vi "Calibration Code for Sonar.vi"() -> ()   [LabVIEW 2014]
uses:
  <vilib>/Instr/_visa.llb/VISA Flush IO Buffer Mask.ctl
  <vilib>/Instr/_visa.llb/VISA Configure Serial Port (Instr).vi
  <vilib>/Utility/file.llb/Read From Spreadsheet File (DBL).vi
panel:
  out "Final Decision Array":dbl[](graph)
  in  "Avg":path
  in  "Min":path
  out "SubFinal Decision Array":dbl[](graph)
  out "Normalized Scan 1":dbl[](graph)
  out "Normalized Scan 2":dbl[](graph)
  out "error out":errorcluster
  out "Done":bool
  out "Position Out":i32
  out "Loop Number":i32
  out "Gauge":i32(knob)
  in  "stop 2":bool
  out "Sensor Head Position 2":i32
  out "THE WHALE IS AT:":i32
  out "Waveform Graph 2":dbl[](graph)
  in  "?":bool
  out "Stop Engaged 2":bool
  out "Blinky Light 2":bool
  out "read buffer 3":string
  out "return count 3":u32
  out "Distance, in 3":dbl
  out "Waveform Chart 4":dbl(graph)
  in  "Max":path
  out "Waveform Graph":dbl[](graph)
  out "error out 2":errorcluster
  in  "Motor Direction":bool
  in  "?":bool
  out "Stop Engaged":bool
  out "Blinky Light":bool
  out "Sensor Head Position":dbl
  out "Sensor Head Dial":dbl(knob) scale=-800.0..800.0
  out "read buffer 2":string
  out "return count 2":u32
  out "Distance, in 2":dbl
  out "Waveform Chart 3":dbl(graph)
  in  "stop":bool
  out "IR Distance Reading":dbl
  out "Find starting position?":bool
  in  "VISA resource name 2":refnum<visa-resource-name>="COM3"
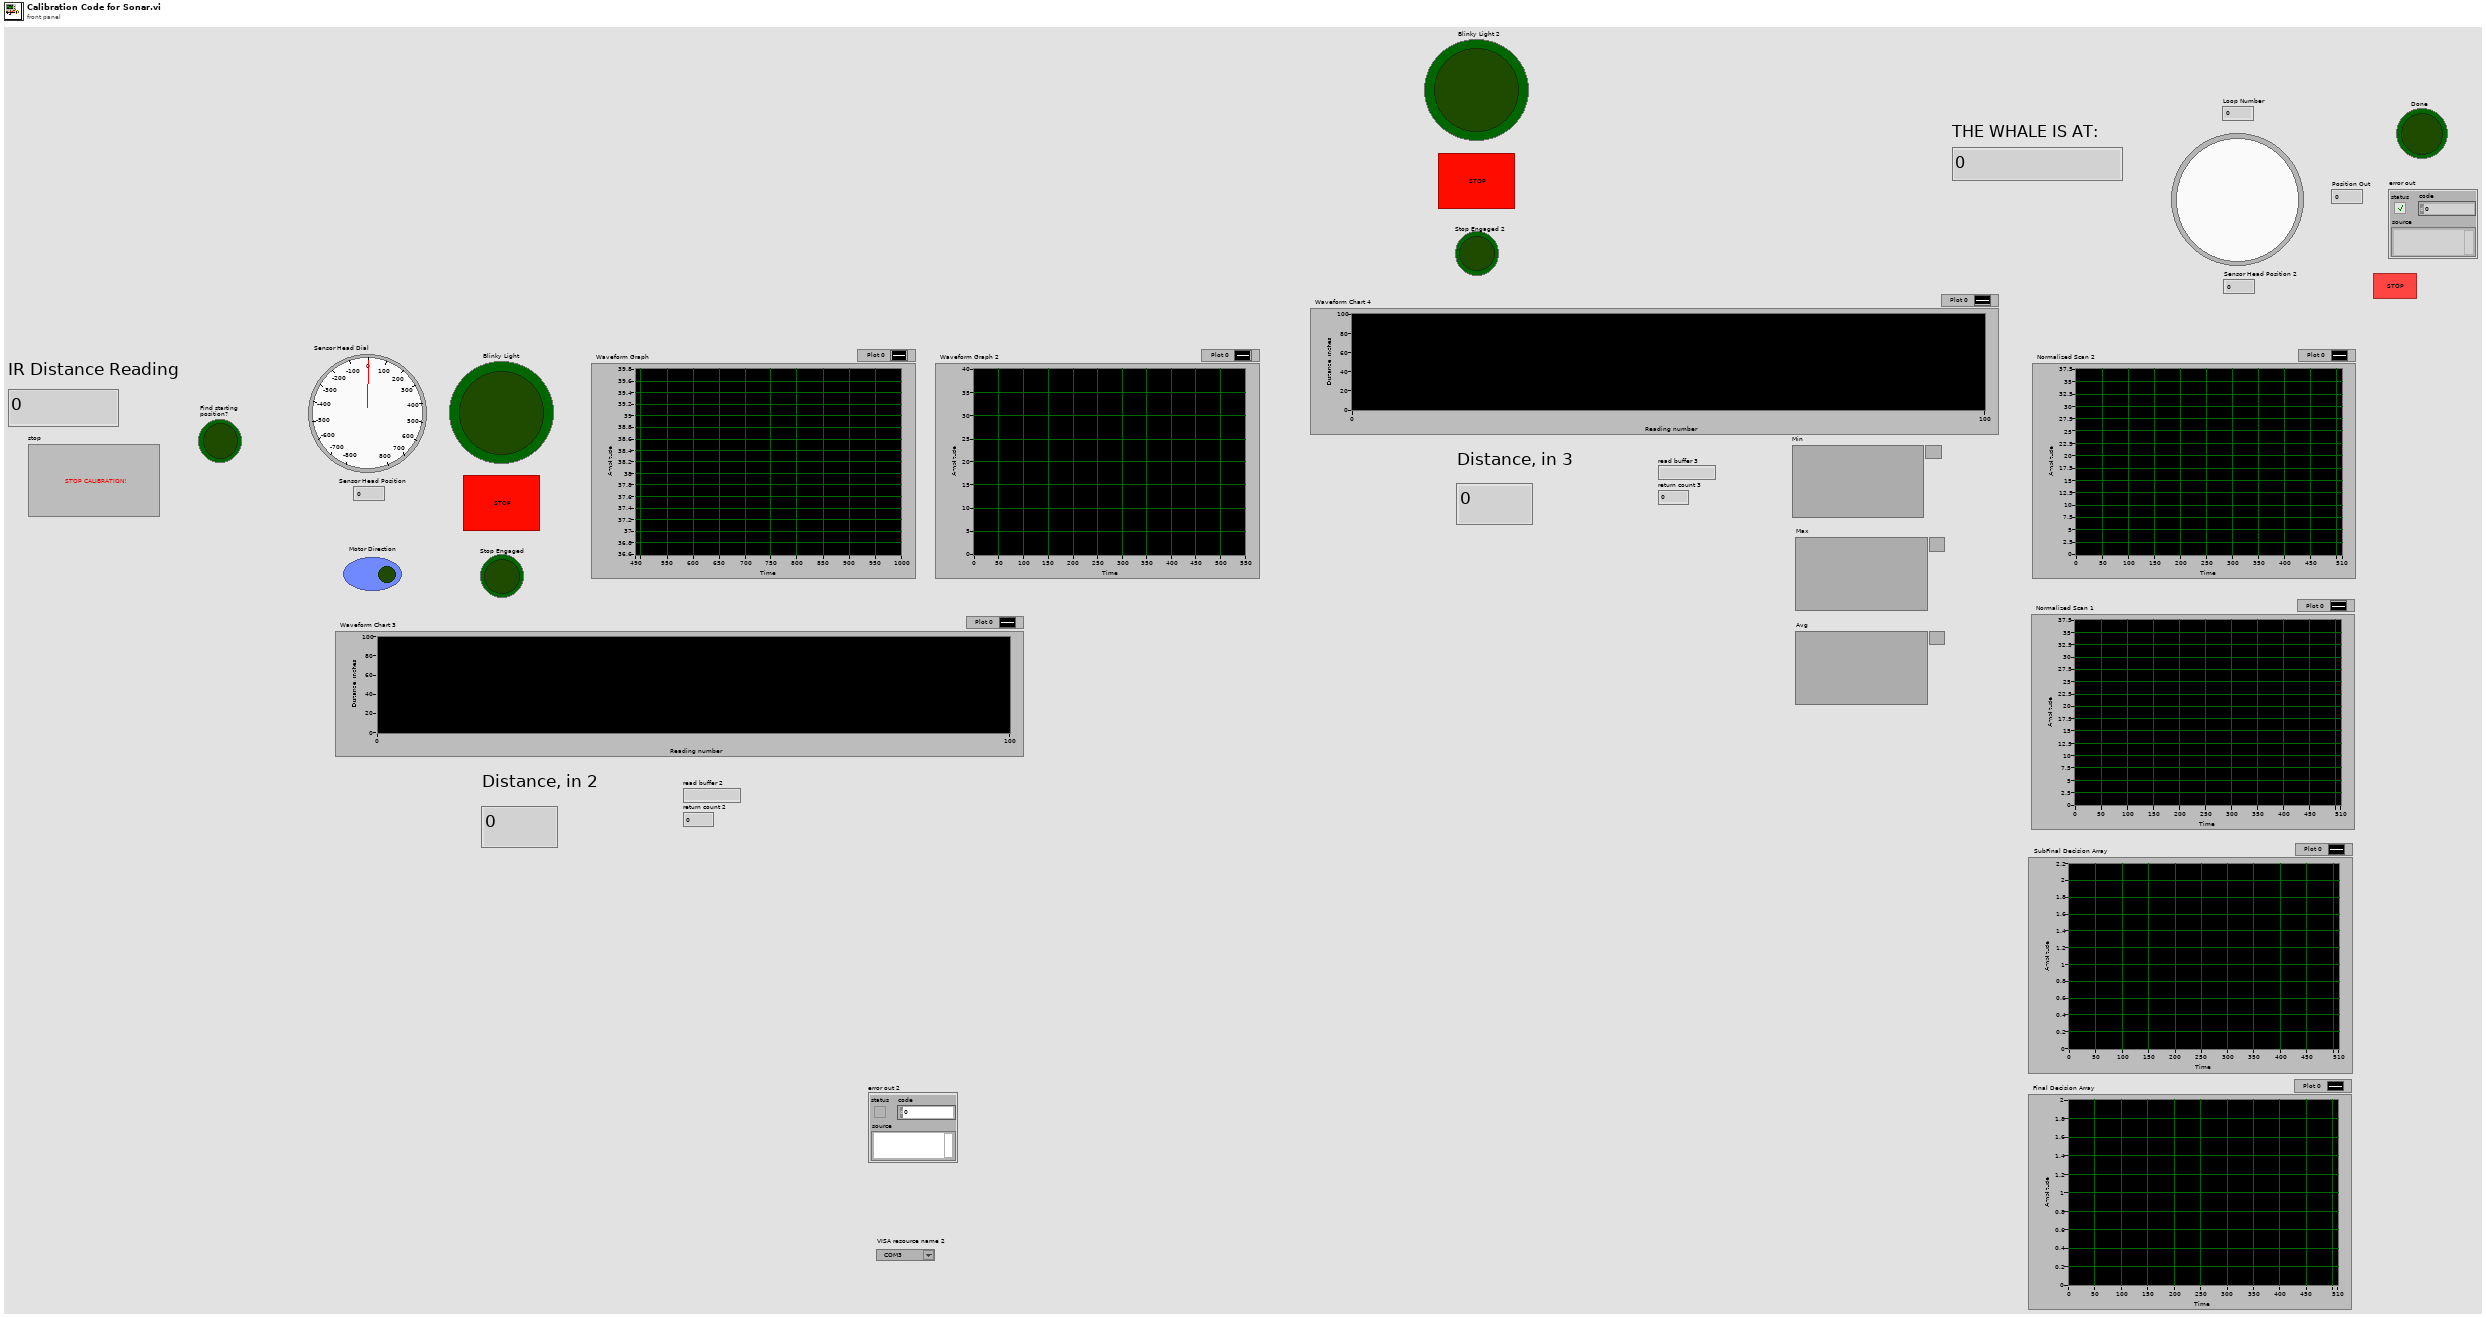
[diagram p1: front panel]
types:
  T1 = typedef "VISA Flush IO Buffer Mask.ctl" = u16
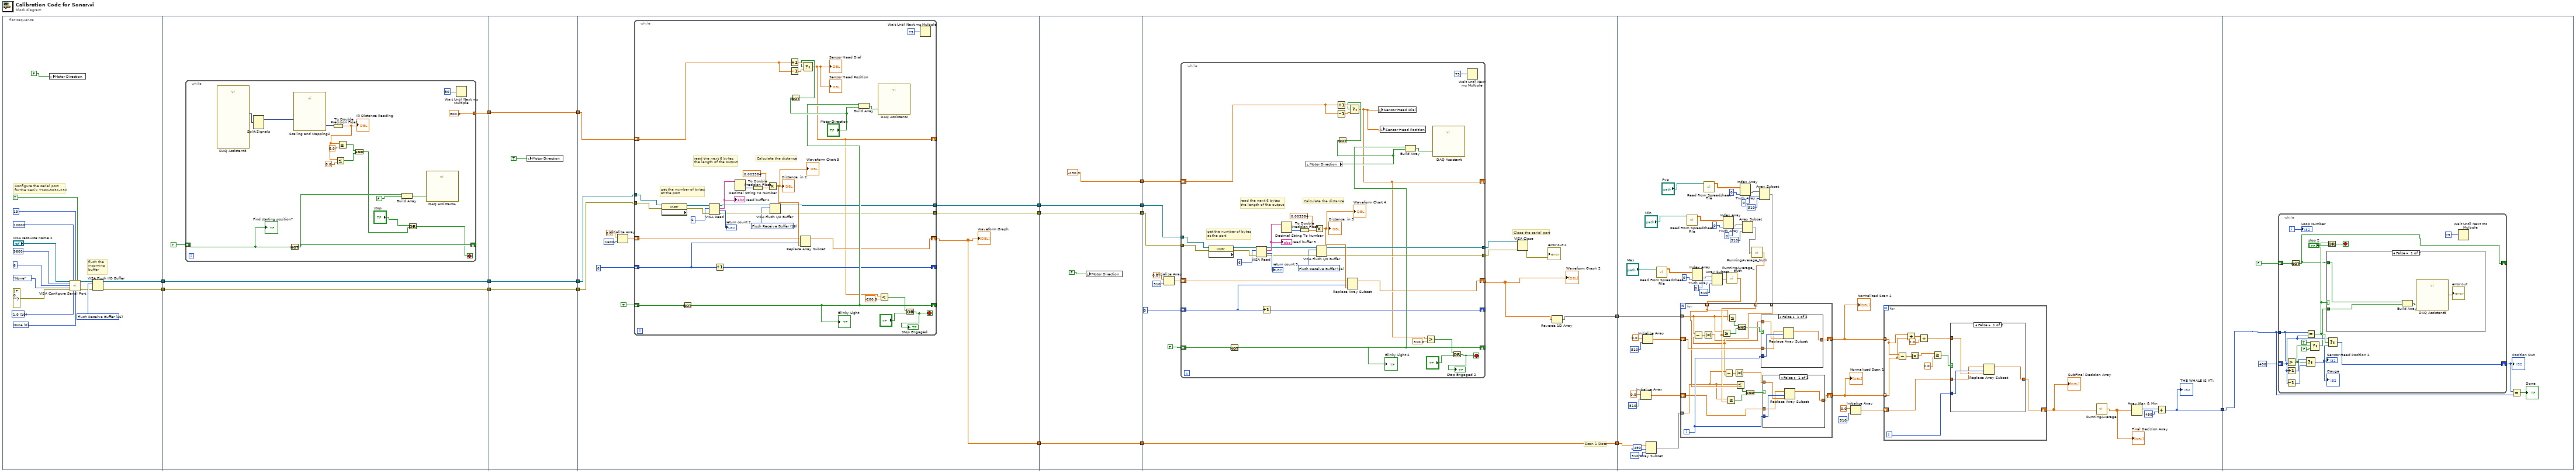
[diagram p0: block diagram]
diagram:
  n1 = flat-sequence {
    tunnel: [w21] -> w18
    tunnel: [w20] -> w17
    tunnel: w18 -> [w38]
    tunnel: w17 -> [w37]
    tunnel: [w35] -> w16
    tunnel: [w38] -> w15
    tunnel: [w37] -> w14
    tunnel: w16 -> [w59]
    tunnel: w15 -> [w58]
    tunnel: w14 -> [w57]
    tunnel: [w59] -> w13
    tunnel: [w58] -> w12
    tunnel: [w57] -> w11
    tunnel: w13 -> [w68]
    tunnel: w12 -> [w67]
    tunnel: w11 -> [w66]
    tunnel: [w62] -> w10
    tunnel: [w61] -> w8
    tunnel: [w60] -> w5
    tunnel: w10 -> [w109]
    tunnel: [w109] -> w9
    tunnel: w8 -> [w108]
    tunnel: [w108] -> w7
    tunnel: [-250.0] -> w6
    tunnel: w5 -> [w105]
    tunnel: [w105] -> w4
    tunnel: w9 -> [w117]
    tunnel: w7 -> [w116]
    tunnel: w6 -> [w115]
    tunnel: w4 -> [w114]
    tunnel: [w114] -> w3
    tunnel: [w110] -> w2
    tunnel: w3 -> [w201]
    tunnel: w2 -> [w199]
    tunnel: [w200] -> w1
    tunnel: w1 -> [w253]
    frame #0 {
      w24 = T1 16 items=["Flush Receive Buffer"=16, "Write Transmit Buffer to Device"=32, "Flush Receive Buffer (No I/O)"=64, "Flush Transmit Buffer"=128] ("Mask")
      w28 = u16 0 items=["None", "XON/XOFF", "RTS/CTS", "XON/XOFF & RTS/CTS", "DTR/DSR", "XON/XOFF & DTR/DSR"] ("flow control (0:none)")
      w30 = u16 10 items=["1.0"=10, "1.5"=15, "2.0"=20] ("stop bits (10: 1 bit)")
      # "flush the \nincoming \nbuffer"
      # "Configure the serial port\nfor the Senix TSPC-3031-232"
      n2 = local write "Motor Direction"(FALSE) -> ()
      n3 = call-poly "VISA Configure Serial Port"("VISA resource name"="VISA resource name 2", "timeout (10sec)"=u32 10000, "termination char\n(0xA = '\\n' = LF)"=u8 13 ("termination char\n(0xA = '\\n' = LF)"), "Enable Termination\nChar (T)"=TRUE ("Enable Termination\nChar (T)"), "baud rate (9600)"=u32 9600, "data bits (8)"=u16 8, "parity (0:none)"=enum16{"None", "Odd", "Even", "Mark", "Space"}."None", "error in (no error)"=errorcluster {"status"=FALSE, "code"=0, "source"=""}, "stop bits (10: 1 bit)"=w30, "flow control (0:none)"=w28) -> ("VISA resource name out"=w23:refnum<visa-resource-name>, "error out"=w22:errorcluster)  [unwired: 4 in]
      n4 = VISA Flush I/O Buffer(VISA resource name=w23, mask (16)=w24, error in (no error)=w22) -> (VISA resource name out=w21:refnum<visa-resource-name>, error out=w20:errorcluster)
    }
    frame #1 {
      n5 = while {
        tunnel: [800.0] -> w35
        shift-right: [w54] -> _
        shift-left: TRUE -> [w52]
        stop <- w41 stop-if-true
        n6 = call "DAQ Assistant3"() -> ("data"=w50:dynamicdata)  [unwired: 16 in, 3 out]
        n7 = Split Signals "Split Signals"(w50) -> (w51:dynamicdata)  [unwired: 5 in, 4 out]
        n8 = Not(x=w52) -> (.not. x?=w54:bool)
        n9 = call "Scaling and Mapping2"("Signals"=w51) -> ("Scaled Signals"=w45:dynamicdata)  [unwired: 9 in, 1 out]
        n10 = To Double Precision Float(number=w45) -> (double precision float=w44:dbl)
        "IR Distance Reading" <- w44
        n11 = Less Or Equal?(x=w44, y=8.0) -> (x <= y?=w46:bool)
        n12 = Greater Or Equal?(x=w44, y=6.0) -> (x >= y?=w47:bool)
        n13 = And(x=w47, y=w46) -> (x .and. y?=w42:bool)
        n14 = Build Array(w54, FALSE) -> (w55:bool[])
        n15 = Or(x="stop", y=w42) -> (x .or. y?=w41:bool)
        n16 = call "DAQ Assistant4"("data"=w55) -> ()  [unwired: 17 in, 2 out]
        n17 = Wait Until Next ms Multiple(millisecond multiple=50) -> ()  [unwired: 1 out]
        "Find starting position?" <- w52
      }
    }
    frame #2 {
      n18 = local write "Motor Direction"(TRUE) -> ()
    }
    frame #3 {
      n19 = Initialize Array(0.0 ("element"), 1600 ("dimension size")) -> (w69:dbl[])
      n20 = while {
        shift-right: [w71] -> _
        shift-left: w68 -> [w101]
        shift-right: [w82] -> _
        shift-left: TRUE -> [w96]
        tunnel: w67 -> [w81]
        tunnel: w66 -> [w80]
        shift-right: [w77] -> w60
        shift-left: w69 -> [w79]
        shift-right: [w76] -> _
        shift-left: 0 ("dimension size") -> [w78]
        tunnel: [w75] -> w61
        tunnel: [w74] -> w62
        stop <- w95 stop-if-true
        w85 = T1 16 items=["Flush Receive Buffer"=16, "Write Transmit Buffer to Device"=32, "Flush Receive Buffer (No I/O)"=64, "Flush Transmit Buffer"=128] ("Mask")
        # "Calculate the distance"
        # "read the next 6 bytes\nthe length of the output"
        # "get the number of bytes\nat the port"
        n21 = property class="Instr" props=["Serial Settings:Number of Bytes at Serial Port"](reference=w81, error in=w80) -> (reference out=w94:refnum<visa-resource-name>, error out=w93:errorcluster)  [unwired: 1 out]
        n22 = Not(x=w96) -> (.not. x?=w82:bool)
        "Blinky Light" <- w82
        n23 = VISA Read(VISA resource name=w94, byte count=u32 6, error in (no error)=w93) -> (VISA resource name out=w87:refnum<visa-resource-name>, read buffer=w91:string, return count=→"return count 2":u32, error out=w86:errorcluster)
        "read buffer 2" <- w91
        n24 = Increment(x=w78) -> (x+1=w76:i32)
        n25 = Decimal String To Number(string=w91) -> (number=w90:i32)  [unwired: 2 in, 1 out]
        n26 = To Double Precision Float(number=w90) -> (double precision float=w89:dbl)
        n27 = Multiply(x=0.003384, y=w89) -> (x*y=w83:dbl)
        "Distance, in 2" <- w83
        "Waveform Chart 3" <- w83
        n28 = VISA Flush I/O Buffer(VISA resource name=w87, mask (16)=w85, error in (no error)=w86) -> (VISA resource name out=w75:refnum<visa-resource-name>, error out=w74:errorcluster)
        n29 = Increment(x=w101) -> (x+1=w103:dbl)
        n30 = Decrement(x=w101) -> (x-1=w102:dbl)
        n31 = Not(x="Motor Direction") -> (.not. x?=w99:bool)
        n32 = Replace Array Subset(array=w79, new element=w83, index=w78) -> (w77:dbl[])
        n33 = Select(t=w103, s=w99, f=w102) -> (s? t:f=w71:dbl)
        "Sensor Head Position" <- w71
        "Sensor Head Dial" <- w71
        n34 = Build Array(w82, "Motor Direction") -> (w97:bool[])
        n35 = call "DAQ Assistant2"("data"=w97) -> ()  [unwired: 17 in, 2 out]
        n36 = Less?(x=w71, y=-200.0) -> (x < y?=w73:bool)
        n37 = Or(x=w73, y="?") -> (x .or. y?=w95:bool)
        "Stop Engaged" <- w95
        n38 = Wait Until Next ms Multiple(millisecond multiple=75) -> ()  [unwired: 1 out]
      }
      "Waveform Graph" <- w60
    }
    frame #4 {
      n39 = local write "Motor Direction"(FALSE) -> ()
    }
    frame #5 {
      # "Scan 1 Data"
      # "Close the serial port"
      n40 = Initialize Array(0.0 ("element"), 510 ("dimension size")) -> (w121:dbl[])
      n41 = while {
        shift-right: [w124] -> _
        shift-left: w115 -> [w154]
        shift-right: [w136] -> _
        shift-left: TRUE -> [w150]
        tunnel: w116 -> [w135]
        tunnel: w117 -> [w134]
        shift-right: [w131] -> w111
        shift-left: w121 -> [w133]
        shift-right: [w130] -> _
        shift-left: 0 ("dimension size") -> [w132]
        tunnel: [w129] -> w113
        tunnel: [w128] -> w112
        stop <- w149 stop-if-true
        w139 = T1 16 items=["Flush Receive Buffer"=16, "Write Transmit Buffer to Device"=32, "Flush Receive Buffer (No I/O)"=64, "Flush Transmit Buffer"=128] ("Mask")
        # "Calculate the distance"
        # "read the next 6 bytes\nthe length of the output"
        # "get the number of bytes\nat the port"
        n42 = property class="Instr" props=["Serial Settings:Number of Bytes at Serial Port"](reference=w135, error in=w134) -> (reference out=w148:refnum<visa-resource-name>, error out=w147:errorcluster)  [unwired: 1 out]
        n43 = Not(x=w150) -> (.not. x?=w136:bool)
        "Blinky Light 2" <- w136
        n44 = VISA Read(VISA resource name=w148, byte count=u32 6, error in (no error)=w147) -> (VISA resource name out=w141:refnum<visa-resource-name>, read buffer=w145:string, return count=→"return count 3":u32, error out=w140:errorcluster)
        "read buffer 3" <- w145
        n45 = Increment(x=w132) -> (x+1=w130:i32)
        n46 = Decimal String To Number(string=w145) -> (number=w144:i32)  [unwired: 2 in, 1 out]
        n47 = To Double Precision Float(number=w144) -> (double precision float=w143:dbl)
        n48 = local read "Motor Direction"() -> (w125:bool)
        n49 = Multiply(x=0.003384, y=w143) -> (x*y=w137:dbl)
        "Distance, in 3" <- w137
        "Waveform Chart 4" <- w137
        n50 = VISA Flush I/O Buffer(VISA resource name=w141, mask (16)=w139, error in (no error)=w140) -> (VISA resource name out=w129:refnum<visa-resource-name>, error out=w128:errorcluster)
        n51 = Increment(x=w154) -> (x+1=w156:dbl)
        n52 = Decrement(x=w154) -> (x-1=w155:dbl)
        n53 = Not(x=w125) -> (.not. x?=w152:bool)
        n54 = Replace Array Subset(array=w133, new element=w137, index=w132) -> (w131:dbl[])
        n55 = Select(t=w156, s=w152, f=w155) -> (s? t:f=w124:dbl)
        n56 = local write "Sensor Head Dial"(w124) -> ()
        n57 = local write "Sensor Head Position"(w124) -> ()
        n58 = Build Array(w136, w125) -> (w151:bool[])
        n59 = Greater?(x=w124, y=310.0) -> (0:w127:bool)
        n60 = call "DAQ Assistant"("data"=w151) -> ()  [unwired: 17 in, 2 out]
        n61 = Or(x=w127, y="?") -> (x .or. y?=w149:bool)
        "Stop Engaged 2" <- w149
        n62 = Wait Until Next ms Multiple(millisecond multiple=75) -> ()  [unwired: 1 out]
      }
      "Waveform Graph 2" <- w111
      n63 = VISA Close(VISA resource name=w113, error in (no error)=w112) -> (error out=→"error out 2":errorcluster)
      n64 = Reverse 1D Array(array=w111) -> (reversed array=w110:dbl[])
    }
    frame #6 {
      n65 = Initialize Array "Initialize Array"(0.0 ("element"), 510 ("dimension size")) -> (w187:dbl[])
      n66 = Initialize Array "Initialize Array"(0.0 ("element"), 510 ("dimension size")) -> (w190:dbl[])
      n67 = Array Subset(array=w201, index=490, length=510) -> (w196:dbl[])
      n68 = call-poly <vilib>:"Read From Spreadsheet File.vi"("file path (dialog if empty)"="Max") -> ("all rows"=w194:dbl[][])  [unwired: 6 in, 4 out]
      n69 = call-poly <vilib>:"Read From Spreadsheet File.vi"("file path (dialog if empty)"="Min") -> ("all rows"=w176:dbl[][])  [unwired: 6 in, 4 out]
      n70 = Index Array "Truth Array"(array=w194, index (col)=0 ("index")) -> (element=w181:dbl[])  [unwired: 1 in]
      n71 = call-poly <vilib>:"Read From Spreadsheet File.vi"("file path (dialog if empty)"="Avg") -> ("all rows"=w170:dbl[][])  [unwired: 6 in, 4 out]
      n72 = Array Subset(array=w181, index=0, length=510) -> (w161:dbl[])
      n73 = Index Array "Truth Array"(array=w176, index (col)=0 ("index")) -> (element=w174:dbl[])  [unwired: 1 in]
      n74 = call "RunningAverage_truth.vi"("Input Decision Array"=w161) -> ("Output Decision Array"=w160:dbl[])
      n75 = Index Array "Truth Array"(array=w170, index (col)=0 ("index")) -> (element=w168:dbl[])  [unwired: 1 in]
      n76 = Array Subset(array=w174, index=0, length=510) -> (w159:dbl[])
      n77 = call "RunningAverage_truth.vi"("Input Decision Array"=w159) -> ("Output Decision Array"=w158:dbl[])
      n78 = Array Subset(array=w168, index=0, length=510) -> (w164:dbl[])
      n79 = for {
        tunnel: w199 -> [w221] mode=indexing
        tunnel: w160 -> [w233] mode=indexing
        shift-right: [w237] -> w178
        shift-left: w190 -> [w238]
        tunnel: w196 -> [w223] mode=indexing
        shift-right: [w234] -> w177
        shift-left: w187 -> [w235]
        tunnel: w158 -> [w232] mode=indexing
        tunnel: w164 -> [w220] mode=indexing
        i -> [w236]
        n80 = Subtract(x=w221, y=w220) -> (x-y=w225:dbl)
        n81 = Absolute Value(x=w225) -> (abs(x)=w219:dbl)
        n82 = Greater Or Equal?(x=w221, y=w232) -> (x >= y?=w229:bool)
        n83 = Subtract(x=w223, y=w220) -> (x-y=w224:dbl)
        n84 = Greater Or Equal?(x=w223, y=w232) -> (x >= y?=w227:bool)
        n85 = Less Or Equal?(x=w221, y=w233) -> (x <= y?=w231:bool)
        n86 = Absolute Value(x=w224) -> (abs(x)=w222:dbl)
        n87 = Less Or Equal?(x=w223, y=w233) -> (x <= y?=w226:bool)
        n88 = And(x=w231, y=w229) -> (x .and. y?=w230:bool)
        n89 = And(x=w226, y=w227) -> (x .and. y?=w228:bool)
        n90 = case shown="False" w230 {
          tunnel: w238 -> [w245 w248]
          tunnel: [w244 w248] -> w237
          tunnel: w219 -> [w246 _]
          tunnel: w236 -> [w247 _]
          frame False {
            n91 = Replace Array Subset "Replace Array Subset"(array=w245, new element=w246, index=w247) -> (w244:dbl[])
          }
          frame True {
          }
        }
        n92 = case shown="False" w228 {
          tunnel: w235 -> [w240 w243]
          tunnel: [w239 w243] -> w234
          tunnel: w222 -> [w241 _]
          tunnel: w236 -> [w242 _]
          frame False {
            n93 = Replace Array Subset "Replace Array Subset"(array=w240, new element=w241, index=w242) -> (w239:dbl[])
          }
          frame True {
          }
        }
      }
      "Normalized Scan 2" <- w178
      "Normalized Scan 1" <- w177
      n94 = Initialize Array "Initialize Array"(0.0 ("element"), 510 ("dimension size")) -> (w184:dbl[])
      n95 = for {
        tunnel: w178 -> [w206] mode=indexing
        tunnel: w177 -> [w205] mode=indexing
        shift-right: [w208] -> w163
        shift-left: w184 -> [w210]
        i -> [w207]
        n96 = Subtract(x=w206, y=w205) -> (x-y=w213:dbl)
        n97 = Add(x=w206, y=w205) -> (x+y=w204:dbl)
        n98 = Absolute Value(x=w213) -> (abs(x)=w211:dbl)
        n99 = Divide(x=w204, y=2.0) -> (x/y=w202:dbl)
        n100 = Greater Or Equal?(x=w211, y=2.0) -> (x >= y?=w209:bool)
        n101 = case shown="False" w209 {
          tunnel: w210 -> [w215 w218]
          tunnel: [w214 w218] -> w208
          tunnel: w207 -> [w217 _]
          tunnel: w202 -> [w216 _]
          frame False {
            n102 = Replace Array Subset "Replace Array Subset"(array=w215, new element=w216, index=w217) -> (w214:dbl[])
          }
          frame True {
          }
        }
      }
      "SubFinal Decision Array" <- w163
      n103 = call "RunningAverage.vi"("Input Decision Array"=w163) -> ("Output Decision Array"=w162:dbl[])
      "Final Decision Array" <- w162
      n104 = Array Max & Min(array=w162) -> (max index (indices)=w183:i32)  [unwired: 3 out]
      n105 = Add(x=w183, y=490) -> (x+y=w200:i32)
      "THE WHALE IS AT:" <- w200
    }
    frame #7 {
      n106 = while {
        shift-right: [w267] -> w251
        shift-left: 490 -> [w264]
        tunnel: w253 -> [w265]
        shift-right: [w254] -> _
        shift-left: FALSE -> [w255]
        i -> [w270]
        stop <- w269 stop-if-true
        n107 = Greater?(x=w265, y=w264) -> (0:w258:bool)
        n108 = Increment(x=w264) -> (x+1=w262:i32)
        n109 = Decrement(x=w264) -> (x-1=w263:i32)
        n110 = Not(x=w255) -> (.not. x?=w254:bool)
        n111 = Select(t=w262, s=w258, f=w263) -> (s? t:f=w257:i32)
        "Gauge" <- w257
        "Sensor Head Position 2" <- w257
        n112 = Equal?(x=w265, y=w264) -> (x = y?=w266:bool)
        n113 = Select(t=TRUE, s=w258, f=FALSE) -> (s? t:f=w259:bool)
        n114 = Or(x=w266, y="stop 2") -> (x .or. y?=w269:bool)
        n115 = case shown="False" w266 {
          tunnel: w259 -> [w272 _]
          tunnel: w254 -> [w271 _]
          frame False {
            n116 = Build Array(w271, w272) -> (w274:bool[])
            n117 = call "DAQ Assistant5"("data"=w274) -> ("error out"=→"error out":errorcluster)  [unwired: 17 in, 1 out]
          }
          frame True {
            # "If Desired = Current, don't step the motor"
          }
        }
        n118 = Select(t=w264, s=w266, f=w257) -> (s? t:f=w267:i32)
        n119 = Wait Until Next ms Multiple(millisecond multiple=75) -> ()  [unwired: 1 out]
        "Loop Number" <- w270
      }
      "Position Out" <- w251
      n120 = Equal?(x=w251, y=w253) -> (x = y?=→"Done":bool)
    }
  }
